vi "传感器数据.vi"() -> (3 "传感器读数":T1 {"工位二扭矩" format="%#.3f"; "工位一扭矩" format="%#.3f"; "工位二编码器位移" format="%#.3f"; "工位一编码器位移" format="%#.3f"; "工位二移载伺服位移" format="%#.3f"; "工位一移载伺服位移" format="%#.3f"; "工位二驱动伺服位移" format="%#.3f"; "工位一驱动伺服位移" format="%#.3f"})   [LabVIEW 2020]
uses:
  Libraries/S7/S7.lvlib
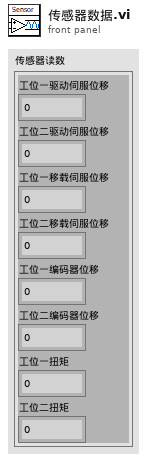
[diagram p1: front panel]
types:
  T1 = cluster{"工位一驱动伺服位移":sgl, "工位二驱动伺服位移":sgl, "工位一移载伺服位移":sgl, "工位二移载伺服位移":sgl, "工位一编码器位移":sgl, "工位二编码器位移":sgl, "工位一扭矩":sgl, "工位二扭矩":sgl}
  T2 = typedef "S7.lvlib/Read_Data (Reply Payload)--cluster.ctl" = cluster{"读取成功":bool, "数据":u32[], "Read_Data_error":errorcluster}
  T3 = cluster{"[0]":sgl, "[1]":sgl, "[2]":sgl, "[3]":sgl, "[4]":sgl, "[5]":sgl, "[6]":sgl, "[7]":sgl}
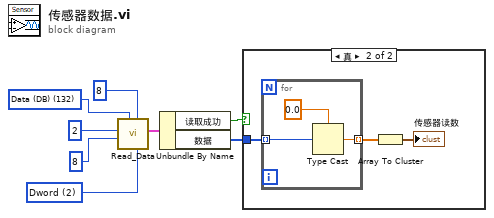
[diagram p0: block diagram]
diagram:
  w5 = u16 2 items=["byte", "word", "Dword"] ("数据类型")
  w6 = u8 132 items=["I/O (P)"=128, "Input (I)"=129, "Output (Q)"=130, "Bit Memory (M)"=131, "Data (DB)"=132, "Instance Data (DI)"=133, "Local Data (L)"=134, "Predecessor Local Data (VL)"=135] ("寄存器类型")
  n1 = call "Read_Data.vi"("数据类型"=w5, "读取长度"=u16 8, "寄存器类型"=w6, "起始地址"=u32 8, "DB #"=u16 2) -> ("Reply Payload"=w3:T2)  [unwired: 4 in, 2 out]
  n2 = Unbundle By Name(w3) -> ("读取成功"=w1:bool, "数据"=w2:u32[])
  n3 = case shown="真" w1 {
    tunnel: w2 -> [_ w11]
    frame False {
    }
    frame True {
      n4 = for {
        tunnel: w11 -> [w13] mode=indexing
        tunnel: [w12] -> w10 mode=indexing
        n5 = Type Cast(type=sgl 0.0, x=w13) -> (*(type *) &x=w12:sgl)
      }
      n6 = Array To Cluster(array=w10) -> (cluster=→"传感器读数":T3)
    }
  }
